vi "test2-LocalExternalStatusRegistrationViaAPI.vi"(8 "error in (no error)":errorcluster, 11 "TestCase in":refnum<class "testcase-CSMStatusStateRegisterUnregister.lvclass">) -> (0 "error out":errorcluster, 3 "TestCase out":refnum<class "testcase-CSMStatusStateRegisterUnregister.lvclass">)   [LabVIEW 2017, in "testcase-CSMStatusStateRegisterUnregister.lvclass"]
uses:
  testcase-CSMStatusStateRegisterUnregister.lvclass
  0b17d103-e67b-41be-a9eb-a2ee1311ff1f.vi
  5999693e-4f8a-4b34-ae87-f34dff5771be.vi
  52a2a10a-a04b-4bad-8df4-e1eb944f47cc.vi
  826f03dd-b4b5-4c6b-9085-8edf6da4f43b.vi
  src/user.lib/_NEVSTOP/Communicable State Machine(CSM)/AdvanceAPI/CSM - Get Module Attribute.vi
  <vilib>/addons/_JKI Toolkits/VI Tester/TestCase.llb/TestCase.lvclass
  src/user.lib/_NEVSTOP/Communicable State Machine(CSM)/Communicable State Machine.lvlib
  C:/Program Files (x86)/National Instruments/LabVIEW 2017/vi.lib/addons/_JKI Toolkits/VI Tester/TestCase.llb/TestCase.lvclass
panel:
  out "LoopCount 2":i32
  out "LoopCount":i32
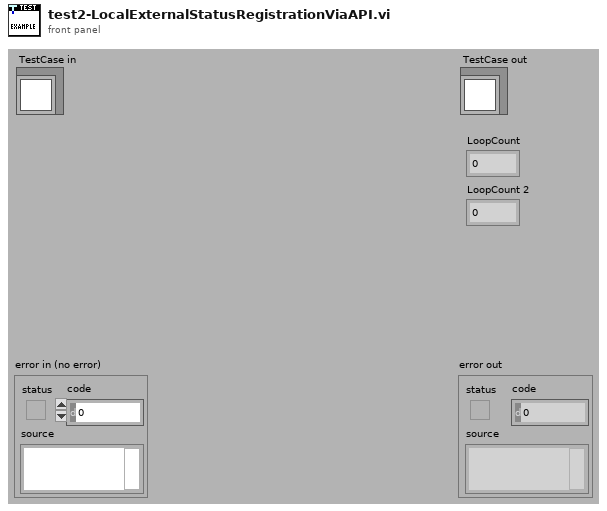
[diagram p1: front panel]
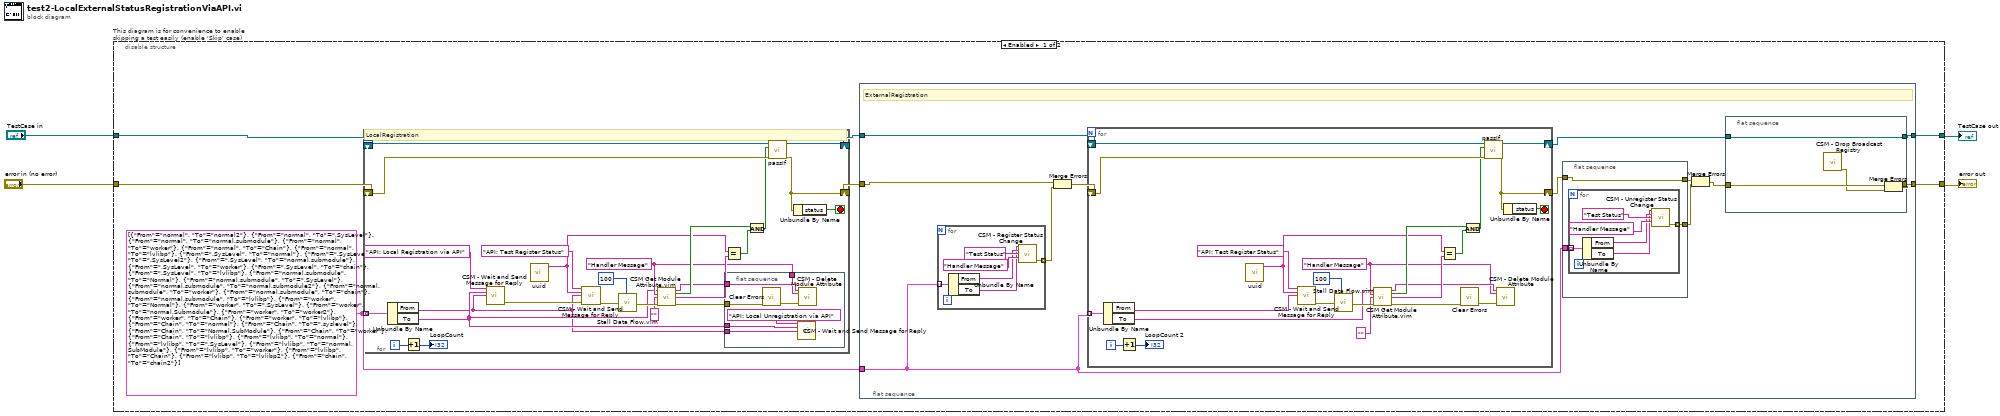
[diagram p0: block diagram]
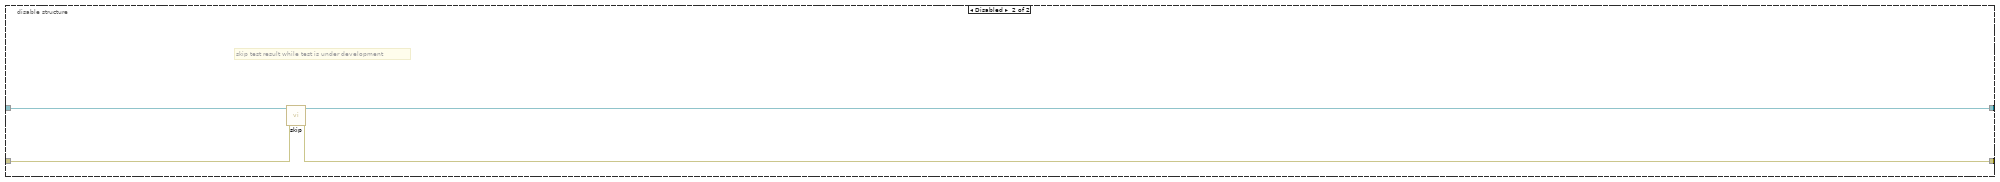
[diagram p2: hidden frame]
diagram:
  n1 = disable-structure "This diagram is for convenience to enable skipping a test easily (enable 'Skip' case)" shown="Enabled" {
    disable-tunnel: "TestCase in" -> [w10 w102]
    disable-tunnel: [w8 w100] -> w1
    disable-tunnel: [w5 w101] -> w3
    disable-tunnel: "error in (no error)" -> [w11 w99]
    frame Enabled {
      w6 = cluster{"From":string, "To":string}[] [{"From"="normal", "To"="normal2"}, {"From"="normal", "To"=".SysLevel"}, {"From"="normal", "To"="normal.submodule"}, {"From"="normal", "To"="worker"}, {"From"="normal", "To"="Chain"}, {"From"="normal", "To"="lvlibp"}, {"From"=".SysLevel", "To"="normal"}, {"From"=".SysLevel", "To"=".SysLevel2"}, {"From"=".SysLevel", "To"="normal.submodule"}, {"From"=".SysLevel", "To"="worker"}, {"From"=".SysLevel", "To"="chain"}, {"From"=".SysLevel", "To"="lvlibp"}, {"From"="normal.submodule", "To"="Normal"}, {"From"="normal.submodule", "To"=".SysLevel"}, {"From"="normal.submodule", "To"="normal.submodule2"}, {"From"="normal.submodule", "To"="worker"}, {"From"="normal.submodule", "To"="chain"}, {"From"="normal.submodule", "To"="lvlibp"}, {"From"="worker", "To"="Normal"}, {"From"="worker", "To"=".SysLevel"}, {"From"="worker", "To"="normal.Submodule"}, {"From"="worker", "To"="worker2"}, {"From"="worker", "To"="Chain"}, {"From"="worker", "To"="lvlibp"}, {"From"="Chain", "To"="normal"}, {"From"="Chain", "To"=".syslevel"}, {"From"="Chain", "To"="Normal.SubModule"}, {"From"="Chain", "To"="worker"}, {"From"="Chain", "To"="lvlibp"}, {"From"="lvlibp", "To"="normal"}, {"From"="lvlibp", "To"=".SysLevel"}, {"From"="lvlibp", "To"="normal.SubModule"}, {"From"="lvlibp", "To"="worker"}, {"From"="lvlibp", "To"="Chain"}, {"From"="lvlibp", "To"="lvlibp2"}, {"From"="chain", "To"="chain2"}]
      n2 = for {
        shift-right: [w20] -> w7
        shift-left: w11 -> [w21]
        shift-right: [w22] -> w9
        shift-left: w10 -> [w23]
        tunnel: w6 -> [w34] mode=indexing
        i -> [w36]
        stop <- w19 stop-if-true
        w14 = "Handler Message" ("To")
        # "LocalRegistration"
        n3 = Unbundle By Name(w34) -> ("From"=w12:string, "To"=w13:string)
        n4 = Increment(x=w36) -> (x+1=→"LoopCount":i32)
        n5 = call "CSM - Wait and Send Message for Reply.vi"("State"="API: Local Registration via API", "Arguments (\"\")"=w13, "Target Module"=w12) -> ("error out"=w31:errorcluster)  [unwired: 10 in, 2 out]
        n6 = call "uuid.vi"() -> ("UUID"=w25:string)  [unwired: 11 in]
        n7 = call "CSM - Wait and Send Message for Reply.vi"("State"="API: Test Register Status", "Arguments (\"\")"=w25, "Target Module"=w12, "Error In (No Error)"=w31) -> ("error out"=w30:errorcluster)  [unwired: 9 in, 2 out]
        n8 = call "Stall Data Flow.vim"("value in"=w30, "milliseconds to wait"=u32 100) -> ("value out"=w28:errorcluster)  [unwired: 1 out]
        n9 = call "CSM Get Module Attribute.vim"("CSM Name"=w13, "Attribute"=w14, "Default Value (Empty Variant)"="", "Error In"=w28) -> ("CSM Name (Dup)"=w15:string, "Found"=w27:bool, "Value"=w24:string, "error out"=w16:errorcluster)  [unwired: 7 in, 1 out]
        n10 = flat-sequence {
          tunnel: w16 -> [w42]
          tunnel: w15 -> [w41]
          tunnel: w14 -> [w40]
          tunnel: w13 -> [w38]
          tunnel: w12 -> [w37]
          frame #0 {
            n11 = call <vilib>:"Clear Errors.vi"("error in (no error)"=w42) -> ("error out"=w43:errorcluster)  [unwired: 5 in, 1 out]
            n12 = call "CSM - Wait and Send Message for Reply.vi"("State"="API: Local Unregistration via API", "Arguments (\"\")"=w38, "Target Module"=w37) -> ()  [unwired: 10 in, 3 out]
            n13 = call "CSM - Delete Module Attribute.vi"("CSM Name"=w41, "Attribute"=w40, "Error In"=w43) -> ()  [unwired: 9 in, 4 out]
          }
        }
        n14 = Equal?(x=w25, y=w24) -> (x = y?=w18:bool)
        n15 = And(x=w27, y=w18) -> (x .and. y?=w17:bool)
        n16 = call-dynamic "passIf.vi"("error in (no error)"=w21, "pass"=w17, "TestCase in"=w23) -> ("error out"=w20:errorcluster, "TestCase out"=w22:refnum<class "testcase-CSMStatusStateRegisterUnregister.lvclass">)  [unwired: 7 in]
        n17 = Unbundle By Name(w20) -> ("status"=w19:bool)
      }
      n18 = flat-sequence {
        tunnel: w9 -> [w55]
        tunnel: [w46] -> w8
        tunnel: w7 -> [w53]
        tunnel: w6 -> [w52]
        tunnel: [w48] -> w5
        frame #0 {
          # "ExternalRegistration"
          n19 = for {
            tunnel: w52 -> [w74] mode=indexing
            tunnel: [w69] -> w50 mode=indexing
            n20 = Unbundle By Name(w74) -> ("From"=w71:string, "To"=w70:string)
            n21 = call "CSM - Register Status Change.vi"("CSM Name"=w70, "Source CSM Name (* as Default)"=w71, "Status"="Test Status", "Response Message (If \"\", Same as Source Message)"="Handler Message" ("Response Message (If \"\", Same as Source Message)")) -> ("error out"=w69:errorcluster)  [unwired: 10 in, 1 out]
          }
          n22 = Merge Errors(w53, w50) -> (w54:errorcluster)
          n23 = for {
            shift-right: [w82] -> w45
            shift-left: w54 -> [w83]
            shift-right: [w84] -> w47
            shift-left: w55 -> [w85]
            tunnel: w52 -> [w96] mode=indexing
            i -> [w98]
            stop <- w81 stop-if-true
            w75 = "Handler Message" ("To")
            n24 = Unbundle By Name(w96) -> ("From"=w94:string, "To"=w90:string)
            n25 = Increment(x=w98) -> (x+1=→"LoopCount 2":i32)
            n26 = call "uuid.vi"() -> ("UUID"=w87:string)  [unwired: 11 in]
            n27 = call "CSM - Wait and Send Message for Reply.vi"("State"="API: Test Register Status", "Arguments (\"\")"=w87, "Target Module"=w94) -> ("error out"=w93:errorcluster)  [unwired: 10 in, 2 out]
            n28 = call "Stall Data Flow.vim"("value in"=w93, "milliseconds to wait"=u32 100) -> ("value out"=w91:errorcluster)  [unwired: 1 out]
            n29 = call "CSM Get Module Attribute.vim"("CSM Name"=w90, "Attribute"=w75, "Default Value (Empty Variant)"="", "Error In"=w91) -> ("CSM Name (Dup)"=w76:string, "Found"=w89:bool, "Value"=w86:string, "error out"=w77:errorcluster)  [unwired: 7 in, 1 out]
            n30 = Equal?(x=w87, y=w86) -> (x = y?=w80:bool)
            n31 = call <vilib>:"Clear Errors.vi"("error in (no error)"=w77) -> ("error out"=w78:errorcluster)  [unwired: 5 in, 1 out]
            n32 = And(x=w89, y=w80) -> (x .and. y?=w79:bool)
            n33 = call-dynamic "passIf.vi"("error in (no error)"=w83, "pass"=w79, "TestCase in"=w85) -> ("error out"=w82:errorcluster, "TestCase out"=w84:refnum<class "testcase-CSMStatusStateRegisterUnregister.lvclass">)  [unwired: 7 in]
            n34 = call "CSM - Delete Module Attribute.vi"("CSM Name"=w76, "Attribute"=w75, "Error In"=w78) -> ()  [unwired: 9 in, 4 out]
            n35 = Unbundle By Name(w82) -> ("status"=w81:bool)
          }
          n36 = flat-sequence {
            tunnel: w52 -> [w58]
            tunnel: [w57] -> w51
            tunnel: w45 -> [w56]
            tunnel: [w56] -> w44
            frame #0 {
              n37 = for {
                tunnel: w58 -> [w64] mode=indexing
                tunnel: [w59] -> w57 mode=indexing
                n38 = Unbundle By Name(w64) -> ("From"=w61:string, "To"=w60:string)
                n39 = call "CSM - Unregister Status Change.vi"("CSM Name"=w60, "Source CSM Name (* as Default)"=w61, "Status"="Test Status", "Response Message (\"*\" as Default)"="Handler Message" ("Response Message (If \"\", Same as Source Message)")) -> ("error out"=w59:errorcluster)  [unwired: 10 in, 1 out]
              }
            }
          }
          n40 = Merge Errors(w44, w51) -> (w49:errorcluster)
          n41 = flat-sequence {
            tunnel: w49 -> [w68]
            tunnel: [w67] -> w48
            tunnel: [w66] -> w46
            tunnel: w47 -> [w66]
            frame #0 {
              n42 = call "CSM - Drop Broadcast Registry.vi"() -> ("error out"=w65:errorcluster)  [unwired: 15 in]
              n43 = Merge Errors(w68, w65) -> (w67:errorcluster)
            }
          }
        }
      }
    }
    frame Disabled {
      # "skip test result while test is under development"
      n44 = call <vilib>:"skip.vi"("error in (no error)"=w99, "TestCase in"=w102) -> ("error out"=w101:errorcluster, "TestCase out"=w100:refnum<class "testcase-CSMStatusStateRegisterUnregister.lvclass">)  [unwired: 8 in]
    }
  }
  "error out" <- w3
  "TestCase out" <- w1
